vi "LJUD_eGetS (DBL Array).vi"(5 "Channel":i32, 7 "IOType":string, 8 "error in":errorcluster, 9 "DBL Array Write":dbl[](array[numeric]) format="%.2f", 10 "Value":i32, 11 "Handle In":i32) -> (0 "error out":errorcluster, 1 "DBL Array Read":dbl[](array[numeric]) format="%.2f", 2 "Value":i32, 3 "Handle Out":i32)   [LabVIEW 2021]
doc: "In this version of eGet the\nIOType is a string. This is a special\nLabVIEW variation of eGetS where\nx1 is declared as a DBL array.\n\nThis is a traditional technique UD\nfunction that internally performs\na single Add, a GoOne, and a single\nGet. See Section 4.1 of the device's\ndatasheet for more information.\n\nIOType specifies what sort of action\nwill be performed. The other inputs\ndepend on the IOType. See the\npseudocode in Section 4.3 for info."
uses:
  labjackud.dll
panel:
  # "This only works for 32-bit.  Use the\nnewer eGetPtr to support 32-bit and\n64-bit.\n\nIn this version of eGet the\nIOType is a string.  This is a special\nLabVIEW variation of eGetS where\nx1 is declared as a DBL array.\n\nThis is a traditional technique UD\nfunction that internally performs\na single Add, a GoOne, and a single\nGet.  See Section 4.1 of the device's\ndatasheet for more information.\n\nIOType specifies what sort of action\nwill be performed.  The other inputs\ndepend on the IOType.  See the\npseudocode in Section 4.3 for info."
  # "Uses \"Reentrant\" for the DLL call."
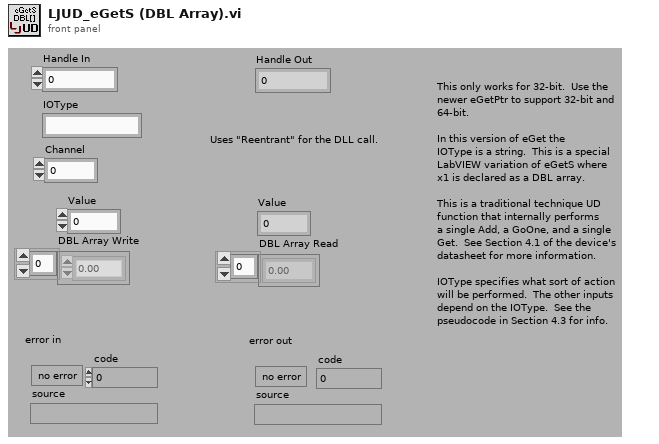
[diagram p1: front panel]
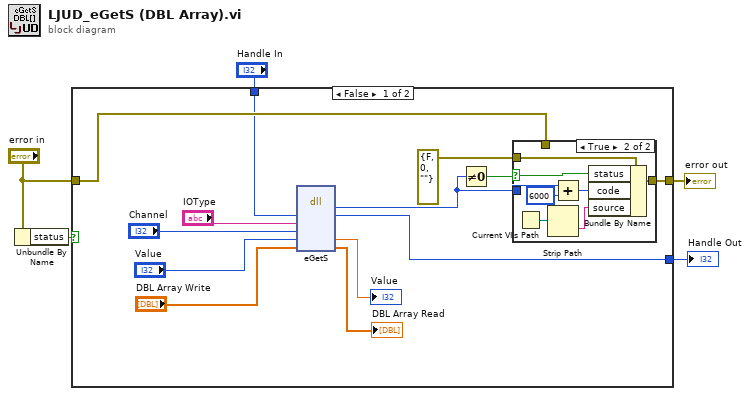
[diagram p0: block diagram]
diagram:
  n1 = Unbundle By Name("error in") -> ("status"=w4:bool)
  n2 = case shown="False" w4 {
    tunnel: [w12 w29] -> w5
    tunnel: "error in" -> [w8 w29]
    tunnel: "Handle In" -> [w7 w28]
    tunnel: [w6 w28] -> w1
    frame False {
      n3 = dll-call lib="labjackud.dll" fn="eGetS"("Handle"=w7, "IOType"="IOType", "Channel"="Channel", "Value"="Value", "x1"="DBL Array Write") -> (w9:i32, "Handle"=w6:i32, "Value"=→"Value":dbl, "x1"=→"DBL Array Read":dbl[])  [unwired: 5 in, 2 out]
      n4 = Not Equal To 0?(x=w9) -> (x != 0?=w10:bool)
      n5 = case shown="True" w10 {
        selector: w10 -> [_ w26]
        tunnel: [w19 w27] -> w12
        tunnel: errorcluster {"status"=FALSE, "code"=0, "source"=""} ("error IO") -> [_ w25]
        tunnel: w9 -> [_ w21]
        tunnel: w8 -> [w19 _]
        frame False {
        }
        frame True {
          n6 = Current VI's Path() -> (path=w23:path)
          n7 = Strip Path(path=w23) -> (name=w24:string)  [unwired: 1 out]
          n8 = Add(x=w21, y=6000) -> (x+y=w22:i32)
          n9 = Bundle By Name(cluster=w25, "status"=w26, "code"=w22, "source"=w24) -> (w27:errorcluster)
        }
      }
    }
    frame True {
    }
  }
  "error out" <- w5
  "Handle Out" <- w1
